vi "Create VariantBuffer.vi"(5 "Buffer":refnum<class "VariantBuffer.lvclass">, 8 "error in":errorcluster, 10 "default":variant, 11 "bufSize":i32) -> (0 "error out":errorcluster, 3 "Buffer":refnum<data-value>)   [LabVIEW 2013, in "VariantBuffer.lvclass"]
doc: "This VI creates a ring buffer of set size. This buffer is created in one place in the memory and is then accessed via pointer/reference.\n\nThe Data Type input is required because it defines the place in the memory to correct size thus removing the need for memory reallocation."
uses:
  VariantBuffer.lvclass
  VariantBuffer.lvclass/VariantBuffer.ctl
panel:
  in  "Allow Overflow? (T)":bool=TRUE
  # "FUTURE USE"
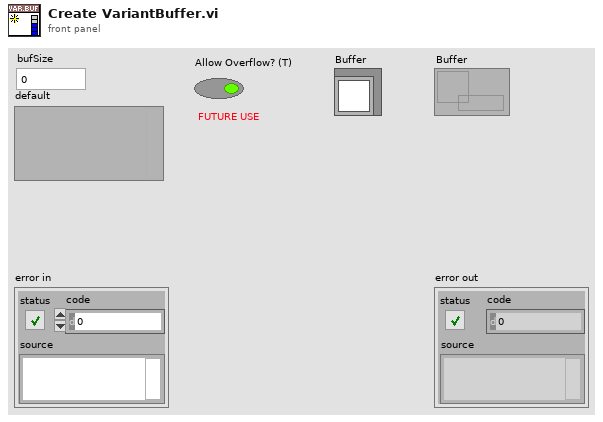
[diagram p1: front panel]
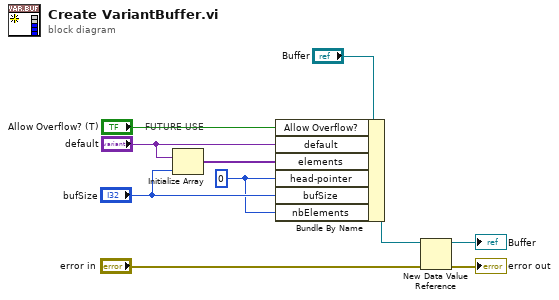
[diagram p0: block diagram]
diagram:
  w3 = 0 ("Index")
  # "FUTURE USE"
  n1 = Initialize Array("default", "bufSize") -> (w9:variant[])
  n2 = Bundle By Name(cluster="Buffer", "Allow Overflow?"="Allow Overflow? (T)", "default"="default", "elements"=w9, "head-pointer"=w3, "bufSize"="bufSize", "nbElements"=w3) -> (w7:refnum<class "VariantBuffer.lvclass">)
  n3 = New Data Value Reference(data value=w7, error in="error in") -> (data value reference=→"Buffer":refnum<data-value>, error out=→"error out":errorcluster)
